vi "After Launch Init.vi"(8 "error in (no error)":errorcluster, 11 "CS++Scope in":refnum<class "CS++Scope.lvclass">) -> (0 "error out":errorcluster, 3 "CS++Scope out":refnum<class "CS++Scope.lvclass">)   [LabVIEW 2014, in "CS++Scope.lvlib" / "CS++Scope.lvclass"]
doc: "Use <b>Pre Launch init.vi</b> method for sanity checks that are supposed to prevent the actor from launching if they fail. Use <B>this</B> method instead to initialize this actor when it has been activated. A corresponding high priority message will become dispatched before the <B>Actor Core.vi</b> is called.\n\n<b>Derived classed should call the parent methode first</b> and their own initialization code after.\n\nRefer also to the ongoing discussion at https://decibel.ni.com/content/message/57394#57394."
uses:
  CS++Scope.lvclass
  CSPP_Core/Classes/CS++ProcessVariables/ProcessVariable/PV.lvclass
  CS++Scope.lvclass/CS++Scope.ctl
  CSPP_Core/Classes/CS++ProcessVariables/ProcessVariable/PV.lvclass/PV.ctl
  <vilib>/ActorFramework/Actor/Actor.lvclass/Actor.ctl
  <vilib>/ActorFramework/Message Enqueuer/Message Enqueuer.lvclass/Message Enqueuer.ctl
  CS++Scope Messages/Configure Acquisition Type Msg/Configure Acquisition Type Msg.lvclass/Configure Acquisition Type Msg.ctl
  CS++Scope Messages/Configure Acquisition Record Msg/Configure Acquisition Record Msg.lvclass/Configure Acquisition Record Msg.ctl
  CS++Scope Messages/Configure Channel Msg/Configure Channel Msg.lvclass/Configure Channel Msg.ctl
  CS++Scope Messages/Configure Trigger Msg/Configure Trigger Msg.lvclass/Configure Trigger Msg.ctl
  CS++Scope Messages/Configure Trigger Modifier [TM] Msg/Configure Trigger Modifier [TM] Msg.lvclass/Configure Trigger Modifier [TM] Msg.ctl
  CS++Scope Messages/Configure Edge Trigger Source Msg/Configure Edge Trigger Source Msg.lvclass/Configure Edge Trigger Source Msg.ctl
  CSPP_Core/Classes/CS++ProcessVariables/ProcessVariable/Write Data.vi
  CSPP_Core/Classes/CS++ProcessVariables/ProcessVariable/Write Error.vi
  CSPP_Core/Classes/CS++ProcessVariables/ProcessVariable/Write Quality.vi
  CSPP_Core/Classes/CS++ProcessVariables/ProcessVariable/Write status.vi
  CSPP_Core/Classes/CS++ProcessVariables/ProcessVariable/Write Timestamp.vi
  <vilib>/ActorFramework/Message Enqueuer/Init from Existing Queue.vi
  <vilib>/ActorFramework/Message Enqueuer/Enqueue.vi
  <vilib>/ActorFramework/Message Priority Queue/Priority Enqueue.vi
  <vilib>/ActorFramework/Message Enqueuer/Message Enqueuer.lvclass
  CS++Scope Messages/Configure Acquisition Type Msg/Configure Acquisition Type Msg.lvclass
  CS++Scope Messages/Configure Acquisition Record Msg/Configure Acquisition Record Msg.lvclass
  CS++Scope Messages/Configure Channel Msg/Configure Channel Msg.lvclass
  CS++Scope Messages/Configure Trigger Msg/Configure Trigger Msg.lvclass
  CS++Scope Messages/Configure Trigger Modifier [TM] Msg/Configure Trigger Modifier [TM] Msg.lvclass
  CS++Scope Messages/Configure Edge Trigger Source Msg/Configure Edge Trigger Source Msg.lvclass
  CSPP_Core/Classes/CS++ProcessVariables/PVConnection/PVConnection.lvclass
  CSPP_Core/Actors/CS++DeviceActor/CS++DeviceActor.lvclass
  <vilib>/ActorFramework/Actor/Actor.lvclass
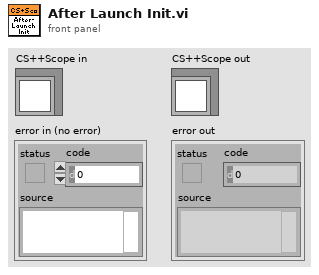
[diagram p1: front panel]
types:
  T1 = cluster{"Write Access":enum8{"Allowed", "Required", "None"}, "Read Access":enum8{"Allowed", "Required", "None"}}
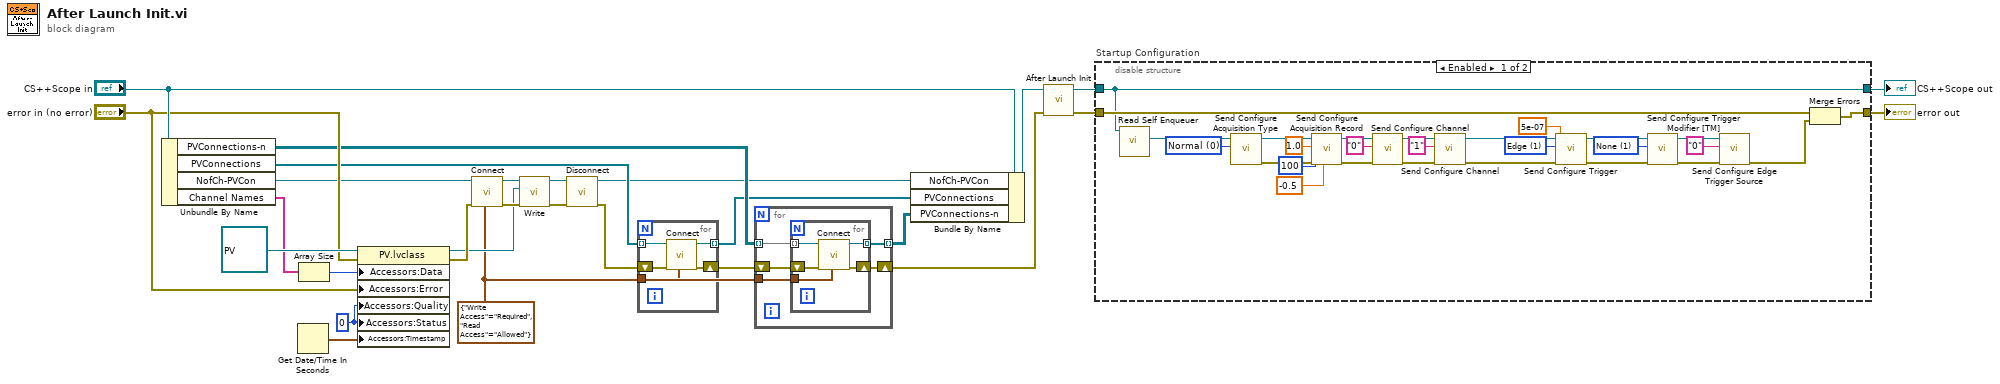
[diagram p0: block diagram]
diagram:
  w8 = 0 ("Status")
  w12 = T1 {"Write Access"=enum."Required", "Read Access"=enum."Allowed"} ("Access (R/W allowed)")
  n1 = Unbundle By Name("CS++Scope in") -> ("PVConnections-n"=w15:refnum<class "PVConnection.lvclass">[][], "PVConnections"=w17:refnum<class "PVConnection.lvclass">[], "NofCh-PVCon"=w24:refnum<class "PVConnection.lvclass">, "Channel Names"=w6:string[])
  n2 = Get Date/Time In Seconds() -> (seconds since 1Jan1904=w7:timestamp)
  n3 = Array Size(array=w6) -> (size(s)=w5:i32)
  n4 = property class="PV.lvclass"(reference=refnum<class "PV.lvclass"> refnum ("CS++ProcessVariables.lvlib:PV.lvclass"), error in="error in (no error)", "Accessors:Data"=w5, "Accessors:Error"="error in (no error)", "Accessors:Quality"=w8, "Accessors:Status"=w8, "Accessors:Timestamp"=w7) -> (reference out=w18:refnum<class "PV.lvclass">, error out=w21:errorcluster)
  n5 = call-dynamic "Connect.vi"("Access (R/W allowed)"=w12, "error in (no error)"=w21, "PVConnection in"=w24) -> ("error out"=w20:errorcluster, "PVConnection out"=w23:refnum<class "PVConnection.lvclass">)  [unwired: 7 in]
  n6 = call-dynamic "Write.vi"("error in (no error)"=w20, "PV"=w18, "PVConnection in"=w23) -> ("error out"=w19:errorcluster, "PVConnection out"=w22:refnum<class "PVConnection.lvclass">)  [unwired: 7 in]
  n7 = call-dynamic "Disconnect.vi"("error in (no error)"=w19, "PVConnection in"=w22) -> ("error out"=w16:errorcluster, "PVConnection out"=w10:refnum<class "PVConnection.lvclass">)  [unwired: 8 in]
  n8 = for {
    tunnel: w17 -> [w33] mode=indexing
    shift-right: [w31] -> w14
    shift-left: w16 -> [w32]
    tunnel: [w30] -> w11 mode=indexing
    tunnel: w12 -> [w29]
    n9 = call-dynamic "Connect.vi"("Access (R/W allowed)"=w29, "error in (no error)"=w32, "PVConnection in"=w33) -> ("error out"=w31:errorcluster, "PVConnection out"=w30:refnum<class "PVConnection.lvclass">)  [unwired: 7 in]
  }
  n10 = for {
    tunnel: w15 -> [w38] mode=indexing
    shift-right: [w36] -> w9
    shift-left: w14 -> [w37]
    tunnel: [w35] -> w13 mode=indexing
    tunnel: w12 -> [w34]
    n11 = for {
      tunnel: w38 -> [w43] mode=indexing
      shift-right: [w41] -> w36
      shift-left: w37 -> [w42]
      tunnel: [w40] -> w35 mode=indexing
      tunnel: w34 -> [w39]
      n12 = call-dynamic "Connect.vi"("Access (R/W allowed)"=w39, "error in (no error)"=w42, "PVConnection in"=w43) -> ("error out"=w41:errorcluster, "PVConnection out"=w40:refnum<class "PVConnection.lvclass">)  [unwired: 7 in]
    }
  }
  n13 = Bundle By Name(cluster="CS++Scope in", "NofCh-PVCon"=w10, "PVConnections"=w11, "PVConnections-n"=w13) -> (w27:refnum<class "CS++Scope.lvclass">)
  n14 = call-parent "After Launch Init.vi"("error in (no error)"=w9, "CS++DeviceActor in"=w27) -> ("error out"=w1:errorcluster, "CS++DeviceActor out"=w2:refnum<class "CS++Scope.lvclass">)  [unwired: 8 in]
  n15 = disable-structure "Startup Configuration" shown="Enabled" {
    disable-tunnel: w1 -> [w70 w71]
    disable-tunnel: [w49 w71] -> w4
    disable-tunnel: [w69 w72] -> w3
    disable-tunnel: w2 -> [w69 w72]
    frame Enabled {
      w61 = 1 items=["None"=1, "Auto"=2, "Auto Level"=3] ("trigger modifier (None)")
      w62 = 1 items=["Edge"=1, "TV"=5, "Runt"=3, "Glitch"=4, "Width"=2, "AC Line"=7, "Immediate"=6] ("trigger type (Edge)")
      w68 = 0 items=["Normal", "Peak Detect", "High Resolution", "Envelope", "Average"] ("acquisition type (Normal)")
      n16 = call <vilib>:"Read Self Enqueuer.vi"("Actor"=w69) -> ("Self Enqueuer"=w60:refnum<class "Message Enqueuer.lvclass">)  [unwired: 10 in]
      n17 = call "Send Configure Acquisition Type.vi"("acquisition type (Normal)"=w68, "Message Enqueuer"=w60) -> ("error out"=w54:errorcluster, "Message Enqueuer out"=w59:refnum<class "Message Enqueuer.lvclass">)  [unwired: 8 in]
      n18 = call "Send Configure Acquisition Record.vi"("acquisition start time (0.0 s)"=dbl[unit] -0.5, "error in (no error)"=w54, "min record length (100 samples)"=100, "time per record (1.0E-3 s)"=dbl[unit] 1.0, "Message Enqueuer"=w59) -> ("error out"=w53:errorcluster, "Message Enqueuer out"=w58:refnum<class "Message Enqueuer.lvclass">)  [unwired: 5 in]
      n19 = call "Send Configure Channel.vi"("error in (no error)"=w53, "channel name (\"CHANNEL1\")"="0" ("channel name (\"CHANNEL1\")"), "Message Enqueuer"=w58) -> ("error out"=w52:errorcluster, "Message Enqueuer out"=w57:refnum<class "Message Enqueuer.lvclass">)  [unwired: 7 in]
      n20 = call "Send Configure Channel.vi"("error in (no error)"=w52, "channel name (\"CHANNEL1\")"="1" ("channel name (\"CHANNEL1\")"), "Message Enqueuer"=w57) -> ("error out"=w51:errorcluster, "Message Enqueuer out"=w56:refnum<class "Message Enqueuer.lvclass">)  [unwired: 7 in]
      n21 = call "Send Configure Trigger.vi"("error in (no error)"=w51, "trigger holdoff (500.0 E-9 s)"=dbl[unit] 5e-07, "trigger type (Edge)"=w62, "Message Enqueuer"=w56) -> ("error out"=w50:errorcluster, "Message Enqueuer out"=w55:refnum<class "Message Enqueuer.lvclass">)  [unwired: 6 in]
      n22 = call "Send Configure Trigger Modifier [TM].vi"("error in (no error)"=w50, "trigger modifier (None)"=w61, "Message Enqueuer"=w55) -> ("error out"=w48:errorcluster, "Message Enqueuer out"=w46:refnum<class "Message Enqueuer.lvclass">)  [unwired: 7 in]
      n23 = call "Send Configure Edge Trigger Source.vi"("error in (no error)"=w48, "trigger source (CHANNEL1)"="0", "Message Enqueuer"=w46) -> ("error out"=w47:errorcluster)  [unwired: 7 in, 1 out]
      n24 = Merge Errors(w70, w47) -> (w49:errorcluster)
    }
    frame Disabled {
    }
  }
  "error out" <- w4
  "CS++Scope out" <- w3
